vi "Read Message (UDP).vi"(8 "error in":errorcluster, 9 "options":T1={"ignore timeout error"=TRUE, "timeout ms (1000)"=1000, "max size (548)"=548}, 11 "connection info in":T3) -> (0 "error out":errorcluster, 1 "name":T4, 2 "data string":string, 3 "connection info out":T3, 4 "data info":T2, 5 "timed out?":bool)   [LabVIEW 2013, in "NI STM.lvlib"]
doc: "This VI reads an incoming package of data from a host. This VI parses the package and extracts the data name and type as described in the meta data.\n\nFor the package to be parsed correctly, the meta data must be consistent in both the sender and the receiver. The data is packaged based on the existing meta data on the sender. \n\nUse the \"STM Read Meta Data\" and \"STM Write Meta Data\" VIs to ensure that both client and server have the same meta data.\n\nThe data is returned as a string. It is the responsibility of the user to cast it to the appropriate type."
uses:
  NI STM.lvlib
  SubVIs/MetaDataElement.ctl
  UDP Connection Info.ctl
  UDP Data Info.ctl
  UDP Read Options.ctl
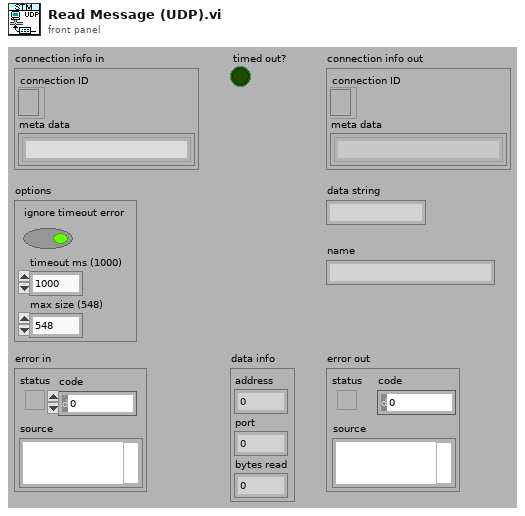
[diagram p1: front panel]
types:
  T1 = typedef "NI STM.lvlib/UDP Read Options.ctl" = cluster{"ignore timeout error":bool, "timeout ms (1000)":i32, "max size (548)":i32}
  T2 = typedef "NI STM.lvlib/UDP Data Info.ctl" = cluster{"address":u32, "port":u16, "bytes read":i32}
  T3 = typedef "NI STM.lvlib/UDP Connection Info.ctl" = cluster{"connection ID":refnum<k16>, "meta data":T4[]}
  T4 = typedef "NI STM.lvlib/MetaDataElement.ctl" = string
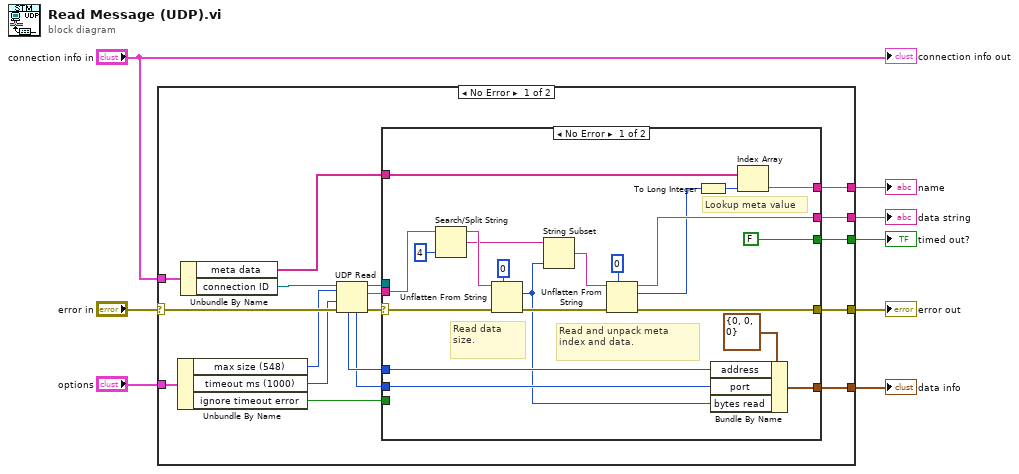
[diagram p0: block diagram]
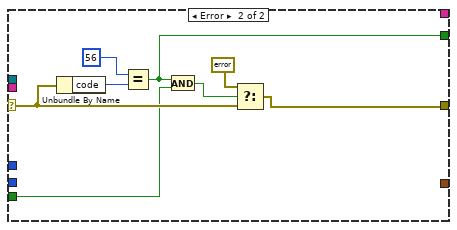
[diagram p2: hidden frame]
diagram:
  n1 = case shown="No Error" "error in" {
    selector: "error in" -> [w17 w56]
    tunnel: "connection info in" -> [w10 _]
    tunnel: [w26 w56] -> w8
    tunnel: [w25 _] -> w7
    tunnel: [w24 _] -> w6
    tunnel: [w23 _] -> w5
    tunnel: "options" -> [w16 _]
    tunnel: [w9 _] -> w2
    frame No Error {
      n2 = Unbundle By Name(w16) -> ("max size (548)"=w14:i32, "timeout ms (1000)"=w13:i32, "ignore timeout error"=w15:bool)
      n3 = Unbundle By Name(w10) -> ("meta data"=w11:T4[], "connection ID"=w12:refnum<k16>)
      n4 = UDP Read(connection ID=w12, max size (548)=w14, timeout ms (25000)=w13, 8:w17) -> (data out=w20:string, error out=w22:errorcluster, 3:w21:refnum<k16>, 4:w18:u16, 6:w19:u32)
      n5 = case shown="No Error" w22 {
        selector: w22 -> [w46 w52]
        tunnel: w20 -> [w40 _]
        tunnel: w21 -> [_ _]
        tunnel: w11 -> [w47 _]
        tunnel: [w45 w51] -> w26
        tunnel: w15 -> [_ w49]
        tunnel: [FALSE w50] -> w25
        tunnel: [w44 _] -> w24
        tunnel: [w35 _] -> w23
        tunnel: w19 -> [w32 _]
        tunnel: w18 -> [w30 _]
        tunnel: [w28 _] -> w9
        frame No Error {
          # "Read data size."
          # "Lookup meta value"
          # "Read and unpack meta index and data."
          n6 = Search/Split String(string=w40, offset (0)=4) -> (substring before match=w39:string, match + rest of string=w38:string)  [unwired: 2 out]
          n7 = Unflatten From String(type=0 ("bytes to read"), binary string=w39, error in (no error)=w46) -> (value=w29:i32, error out=w42:errorcluster)  [unwired: 1 in, 2 out]
          n8 = String Subset(string=w38, length (rest)=w29) -> (substring=w37:string)  [unwired: 1 out]
          n9 = Unflatten From String(type=u16 0, binary string=w37, error in (no error)=w42) -> (rest of the binary string=w35:string, value=w33:u16, error out=w45:errorcluster)  [unwired: 2 out]
          n10 = To Long Integer(number=w33) -> (32bit integer=w34:i32)
          n11 = Bundle By Name(cluster=T2 {"address"=0, "port"=0, "bytes read"=0} ("Data Info"), "address"=w32, "port"=w30, "bytes read"=w29) -> (w28:T2)
          n12 = Index Array(array=w47, index=w34) -> (element=w44:T4)
        }
        frame Error {
          n13 = Unbundle By Name(w52) -> ("code"=w53:i32)
          n14 = Equal?(x=56 ("code"), y=w53) -> (x = y?=w50:bool)
          n15 = And(x=w50, y=w49) -> (x .and. y?=w54:bool)
          n16 = Select(t=errorcluster {"status"=FALSE, "code"=0, "source"=""} ("error out"), s=w54, f=w52) -> (s? t:f=w51:errorcluster)
        }
      }
    }
    frame Error {
    }
  }
  "error out" <- w8
  "timed out?" <- w7
  "data string" <- w5
  "name" <- w6
  "data info" <- w2
  "connection info out" <- "connection info in"
